vi "ComplexMultiplySGL_src.vi"(5 "X":T1, 7 "Y":T1) -> (8 "Z":T1)   [LabVIEW 2015]
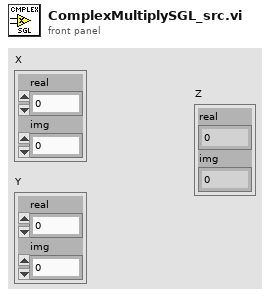
[diagram p1: front panel]
types:
  T1 = typedef "ComplexSGL" = cluster{"real":sgl, "img":sgl}
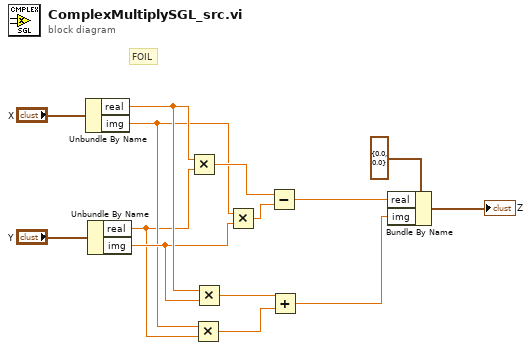
[diagram p0: block diagram]
diagram:
  # "FOIL"
  n1 = Unbundle By Name("X") -> ("real"=w10:sgl, "img"=w7:sgl)
  n2 = Unbundle By Name("Y") -> ("real"=w6:sgl, "img"=w9:sgl)
  n3 = Multiply(x=w10, y=w6) -> (x*y=w12:sgl)
  n4 = Multiply(x=w7, y=w6) -> (x*y=w5:sgl)
  n5 = Multiply(x=w10, y=w9) -> (x*y=w8:sgl)
  n6 = Multiply(x=w7, y=w9) -> (x*y=w11:sgl)
  n7 = Subtract(x=w12, y=w11) -> (x-y=w3:sgl)
  n8 = Add(x=w8, y=w5) -> (x+y=w2:sgl)
  n9 = Bundle By Name(cluster=T1 {"real"=0.0, "img"=0.0} ("Z"), "real"=w3, "img"=w2) -> (→"Z":T1)
